vi "5785 Generation.vi"(11 "Frequency (Hz)":dbl=100000000.0 format="%#_6p") -> (0 "error out":errorcluster)   [LabVIEW 2019]
uses:
  <vilib>/userDefined/Silver/nirio_resource_slv.ctl
  <instrlib>/FlexRIO/API/Host/v1/NI FlexRIO/API/Reference Clock Source.ctl
  Common/Original 5785 Example/Host/Upconversion Mode.ctl
  <instrlib>/FlexRIO/API/Host/v1/NI FlexRIO/API/Configure Reference Clock.vi
  <instrlib>/FlexRIO/API/Host/v1/NI FlexRIO/API/Get Property Reference - Fpga Small.vi
  <instrlib>/FlexRIO/API/Host/v1/NI FlexRIO/API/Configure Analog Start Trigger.vi
  <instrlib>/FlexRIO/API/Host/v1/NI FlexRIO/API/Configure Digital Edge Start Trigger.vi
  <instrlib>/FlexRIO/API/Host/v1/NI FlexRIO/API/Configure Immediate Start Trigger.vi
  <vilib>/measure/matone.llb/Extract Single Tone Information N Chan.vi
  <vilib>/measure/maspectr.llb/FFT Power Spectrum and PSD for N Chan.vi
  <vilib>/FPGAPlugInAG/Dynamic/niLvFpga_Close_Dynamic.vi
  <vilib>/rvi/interface/nirviCloseFPGA/nirviCloseFPGA.xnode
  <instrlib>/FlexRIO/API/Host/v1/NI FlexRIO API v1.lvlib
  <resource>/objmgr/niflexrioapiStream.rc
  <vilib>/measure/NI_MAPro.lvlib
  Common/Original 5785 Example/Host/GettingStarted_5785_Host.lvlib
  <instrlib>/FlexRIO/API/Host/v1/NI FlexRIO/API/Read Stream 1D WDT.vi
panel:
  in  "DUC Freq Shift (Hz)":dbl format="%#_4p"
  in  "DDC Freq Shift (Hz)":dbl format="%#_4p"
  in  "IQ Enabled":bool
  in  "DDC Enabled":bool
  in  "processing mode":T1=enum."None, Two Channels"
  out "AO num Samples":i32=160
  in  "waveform config":T2(array[cluster])=[{"Frequency (Hz)"=500000000.0, "Amplitude (V)"=0.2, "Phase (Deg)"=0.0}, {"Frequency (Hz)"=500000000.0, "Amplitude (V)"=0.20000000000000004, "Phase (Deg)"=0.0}] {"Phase (Deg)" format="%.2p"; "Amplitude (V)" format="%0.2p"; "Frequency (Hz)" format="%0.2p"}
  in  "reference clock source":T3 items=["Default", "Onboard", "PXI_Clk10", "External", "None", "Baseboard Reference"]
  in  "Update Waveform":bool caption="Download AO Waveforms"
  out "Sample Rate":dbl=3200000000.0 format="%#_6p"
  in  "ADC Interleaving Factor":i32=1 min=0 max=2 step=1
  in  "AI num samples":u64=320 step=32
  in  "AI channels":string="AI0,AI1"
  out "Device Power":dbl(slide)=32.59 scale=-1.0..58.0 scale format="%#_3p"
  out "FPGA Temperature":dbl(slide)=48.0 scale=0.0..100.0 scale format="%#_3p"
  in  "Trigger Type":enum32{"Immediate", "Analog", "Digital"}(tab)
  in  "trigger channel":string="AI0"
  in  "rising edge?":bool=TRUE
  in  "level (V)":dbl format="%#_3p"
  in  "hysteresis (V)":dbl=0.01 format="%#_3p"
  in  "digital trigger source":string(combo)
  in  "stop":bool
  in  "Bitfile path":path=path "C:/Repos/bsherman-sandbox/CogRF/5785 Measurements/Common/Original 5785 Example/FPGA Bitfiles/PXIe_5785_KU060.lvbitx"
  in  "Waveform Tab Control":T4(tab)
  out "Waveform Graph":waveform(dbl)[](graph)=[{"t0"=timestamp(0 s since 1904-01-01), "dt"=3.125e-10, "Y"=array[320 elements]}, {"t0"=timestamp(0 s since 1904-01-01), "dt"=3.125e-10, "Y"=array[320 elements]}]
  out "FFT":cluster{"f0":dbl, "df":dbl, "magnitude":dbl[]}[](graph)=[{"f0"=0.0, "df"=10000000.0, "magnitude"=[-82.80063413529373, -79.42075070514161, -79.66654847580517, -84.51801585564033, -82.30375380409255, -84.06983083569486, -85.66588756329017, -81.93454044371977, -82.7334518284433, -90.8972761146736, -87.61278142747294, -104.61353149769258, -96.28538776427862, -95.10865239905246, -100.56521482666498, -91.42478181315082, -87.70246288546254, -96.15482624965125, -83.85755926546608, -89.20973033468074, -90.22419818568508, -98.99668681361555, -98.60506381140829, -93.29284897866715, -83.85257693765564, -82.90006467726401, -83.45941426572493, -80.25008158521148, -79.93161770011034, -79.54616931592298, -81.30831360852552, -89.3926211554797, -85.88224547986444, -82.87485908353914, -81.93656330640073, -79.20811557500818, -79.33127118879915, -83.00000028590416, -90.00021633457037, -88.94291208193506, -94.81520575658656, -89.72483865287286, -90.03506772196766, -88.10479845296439, -84.61607135685057, -84.72807586779753, -82.3263452971978, -82.71547656878712, -95.58083173506547, -88.61789584075763, -86.68540478159909, -83.07923596382108, -82.7659009857978, -91.87050343873932, -84.66676602771557, -79.67758660366972, -79.03719798485804, -86.91335832284452, -99.97611534229983, -92.79230181046542, -87.01921960736439, -83.08071759168135, -83.5536303116052, -91.69363274102763, -88.41514807099949, -84.10637487787747, -82.44488027320298, -85.08159037151373, -86.04882507196643, -90.13991844124908, -94.82822338029456, -97.06431232929042, -99.63177607215952, -87.79637869645369, -90.10079393416046, -91.82607525621145, -92.62007187200066, -97.8504266754619, -86.1258854333692, -86.25934378904303, -102.59108879099308, -90.0771213920622, -82.32664139003381, -80.78431775305042, -91.50907884320321, -87.95306054419447, -85.57843269559798, -93.04673637457378, -83.30460156673297, -82.19833423896098, -83.5215038947126, -96.02648947107404, -87.65556995900711, -84.70085134292157, -88.22032498756884, -103.07939027252586, -108.02210671738155, -86.99055305132113, -88.32179529969324, -90.31615125476408, -84.97901674920863, -83.09883311475267, -84.95671844316507, -85.53395021586064, -90.81842173967111, -93.68611641670468, -84.452817075586, -79.89507522416633, -81.39102595505449, -81.52404503339568, -80.48337477433137, -87.87345095289177, -84.30670527149636, -83.09195779094782, -84.84695356438543, -91.72645233073027, -88.3626801362871, -90.81004429684762, -87.45943061943689, -90.26039906388364, -90.45094731656192, -87.51778499753328, -80.36998792980968, -80.90573377879318, -93.04936796269288, -86.4132138459746, -93.72990076985027, -83.6736250082015, -83.99855859467331, -89.3953164516118, -83.81187005387955, -87.49573067759147, -84.23606489302381, -83.16298492778144, -87.1194948264914, -90.99142642379402, -93.24764967458385, -88.63527313931499, -102.49413654042559, -90.66118161659553, -92.25646188435081, -80.9110366436795, -83.55380603169064, -81.01720552981077, -84.3777210205706, -90.31462939121568, -98.00294051178642, -95.60338217280496, -96.72557339603003, -85.0751852630811, -82.8903033043814, -96.97498517828193, -84.68377849718097, -81.38086551188258, -85.79249998005481, -87.70913834096886, -93.06972137639319, -97.21572279595078, -95.86294146140558, -83.02562226491523]}, {"f0"=0.0, "df"=10000000.0, "magnitude"=[-64.78931072488608, -67.73528418446969, -87.87073015272404, -81.21018837283968, -80.84885582450725, -84.81155481886637, -87.62283168377273, -82.75665314945999, -83.33624895976874, -85.00935247454665, -90.01344899655619, -85.4168344363582, -93.77738192601578, -88.78723575716211, -80.89555662638084, -77.40445430057734, -83.04964925849828, -92.69503327640547, -85.33098178751953, -84.21675735932456, -94.4286131086485, -84.18522106861258, -84.126502324857, -86.19640568640202, -87.43382048150457, -90.03983448655742, -83.08248688320506, -77.13727685427946, -78.52531931117574, -82.27551749332419, -87.38788534435882, -86.09983091368706, -85.9317566084158, -93.3787076269555, -90.43872921677129, -85.03312454760936, -93.48170429395404, -96.606174398692, -84.54369527641475, -80.1677671442906, -82.28530110524787, -83.58711730195151, -82.75878126450083, -83.35504507620462, -86.06919066007586, -101.11499708979125, -91.71195220747622, -83.56465114361383, -79.52150767688725, -79.96380630019732, -91.4050434521125, -83.48310537201712, -81.73837395801057, -87.51107955857, -89.7119800165195, -81.42579926328145, -79.58251225051853, -83.06097697370845, -88.76806290183217, -82.58018678115121, -80.02121778615148, -82.16358703095486, -86.62565282274939, -99.28526757279388, -94.99464094911238, -90.72589358589816, -88.18693112559416, -79.36875927098997, -79.20171789778858, -83.94202736003771, -105.55799216649051, -83.12357738578754, -82.44879182647495, -86.27524307450246, -88.28406841938097, -81.19621273977118, -83.87578114234637, -88.5269238392554, -84.41995093103635, -85.35505706638736, -84.92519624410147, -81.97290731818995, -82.8267656339678, -82.54032928873265, -86.79451163672385, -88.78654921566789, -81.32210725089064, -82.90482422458243, -86.60048725134602, -86.831633705738, -85.73730495943633, -83.52042201274215, -88.5297416330032, -95.45249595410544, -97.22152770134748, -96.95556150404856, -88.61342235545409, -87.4643325338421, -80.28275240840776, -78.03157534185394, -82.88175719417588, -93.39877945578407, -99.90212582359797, -85.2979962460108, -86.22850917558934, -86.56007545671977, -106.08884169104671, -85.38285757853984, -88.82365520443673, -95.23608231604402, -88.02164481094161, -93.28020634203888, -95.02500522087377, -86.86550910566638, -106.28569332849621, -94.87588536988524, -99.26453951216462, -87.13456076973338, -81.47213984719738, -78.75854685696707, -78.65463828489014, -82.49223582204748, -97.5364174442158, -95.08344525435209, -87.23974238111994, -90.45342808286607, -93.02309157165219, -87.82563643069052, -89.6611716765326, -81.02521384215505, -82.27408401978239, -86.2519183286075, -87.26967132350863, -82.01085019692505, -80.81243914798475, -82.27515501657854, -86.70178876516077, -79.23742538829981, -79.68471508937189, -84.67318859876387, -82.27227290640813, -76.20448461790832, -78.88688649209806, -90.59786677274529, -92.25114985663237, -91.460612834368, -91.26343664898255, -82.08959989225445, -86.11895874760603, -95.1222735792313, -86.44672739810025, -78.83968447685616, -79.23597642096348, -87.541546971985, -88.11663602685513, -84.13844747103789, -85.96460534965021, -88.21924098304329, -84.25148312866752, -76.29493493073782]}] caption="Waveform Graph"
  out "detected frequencies":dbl[](array[numeric])=[555552707.7834543, 1412702117.9341562] format="%_4p"
  out "AO Out":waveform(dbl)[](graph)=[{"t0"=timestamp(0 s since 1904-01-01), "dt"=3.125e-10, "Y"=[0.0, 0.16629392246050906, 0.1847759065022574, 0.03901806440322561, -0.1414213562373095, -0.19615705608064604, -0.07653668647301802, 0.11111404660392049, 0.2, 0.11111404660392035, -0.07653668647301787, -0.19615705608064607, -0.14142135623730956, 0.03901806440322578, 0.18477590650225734, 0.16629392246050892, 0.0, -0.16629392246050909, -0.18477590650225734, -0.03901806440322547, 0.14142135623730956, 0.196157056080646, 0.07653668647301785, -0.11111404660392055, -0.19999999999999996, -0.11111404660392023, 0.07653668647301798, 0.19615705608064604, 0.1414213562373094, -0.03901806440322589, -0.18477590650225728, -0.1662939224605088, 5.551115123125783e-17, 0.16629392246050909, 0.18477590650225723, 0.03901806440322533, -0.14142135623730945, -0.19615705608064585, -0.07653668647301788, 0.11111404660392057, 0.1999999999999999, 0.11111404660392012, -0.07653668647301798, -0.196157056080646, -0.14142135623730936, 0.03901806440322589, 0.18477590650225725, 0.16629392246050878, -2.7755575615628914e-17, -0.16629392246050906, -0.18477590650225725, -0.03901806440322536, 0.14142135623730942, 0.19615705608064593, 0.07653668647301794, -0.11111404660392066, -0.1999999999999999, -0.11111404660392014, 0.07653668647301792, 0.19615705608064604, 0.14142135623730945, -0.039018064403225916, -0.18477590650225728, -0.1662939224605088, 0.0, 0.16629392246050914, 0.18477590650225728, 0.03901806440322533, -0.14142135623730945, -0.19615705608064596, -0.07653668647301792, 0.11111404660392063, 0.1999999999999999, 0.11111404660392017, -0.07653668647301792, -0.1961570560806461, -0.14142135623730945, 0.039018064403226, 0.18477590650225728, 0.1662939224605088, 0.0, -0.1662939224605092, -0.18477590650225728, -0.039018064403225305, 0.14142135623730945, 0.196157056080646, 0.07653668647301792, -0.11111404660392071, -0.1999999999999999, -0.11111404660392012, 0.07653668647301792, 0.19615705608064615, 0.14142135623730945, -0.039018064403226055, -0.18477590650225728, -0.1662939224605088, 0.0, 0.16629392246050925, 0.18477590650225728, 0.039018064403225305, -0.14142135623730945, -0.19615705608064601, -0.07653668647301792, 0.11111404660392074, 0.1999999999999999, 0.11111404660392014, -0.07653668647301792, -0.1961570560806461, -0.14142135623730945, 0.03901806440322597, 0.18477590650225728, 0.1662939224605088, 0.0, -0.16629392246050914, -0.18477590650225728, -0.03901806440322539, 0.14142135623730945, 0.196157056080646, 0.07653668647301792, -0.1111140466039206, -0.1999999999999999, -0.11111404660392023, 0.07653668647301792, 0.19615705608064604, 0.14142135623730945, -0.03901806440322583, -0.18477590650225728, -0.16629392246050886, 0.0, 0.16629392246050909, 0.18477590650225728, 0.03901806440322539, -0.14142135623730945, -0.19615705608064593, -0.07653668647301792, 0.1111140466039206, 0.1999999999999999, 0.11111404660392019, -0.07653668647301792, -0.19615705608064607, -0.14142135623730945, 0.039018064403225944, 0.18477590650225728, 0.1662939224605088, 0.0, -0.16629392246050914, -0.18477590650225728, -0.03901806440322533, 0.14142135623730945, 0.19615705608064596, 0.07653668647301792, -0.11111404660392063, -0.1999999999999999, -0.11111404660392017, 0.07653668647301792, 0.1961570560806461, 0.14142135623730945, -0.039018064403226, -0.18477590650225728, -0.1662939224605088]}, {"t0"=timestamp(0 s since 1904-01-01), "dt"=3.125e-10, "Y"=[0.0, 0.16629392246050909, 0.1847759065022574, 0.03901806440322561, -0.1414213562373095, -0.19615705608064612, -0.07653668647301798, 0.11111404660392046, 0.20000000000000004, 0.11111404660392046, -0.076536686473018, -0.19615705608064612, -0.1414213562373095, 0.03901806440322561, 0.1847759065022574, 0.1662939224605091, 0.0, -0.166293922460509, -0.1847759065022574, -0.03901806440322575, 0.1414213562373095, 0.1961570560806461, 0.07653668647301802, -0.11111404660392044, -0.2, -0.11111404660392044, 0.07653668647301787, 0.1961570560806461, 0.14142135623730956, -0.03901806440322575, -0.18477590650225734, -0.16629392246050897, 0.0, 0.16629392246050903, 0.18477590650225734, 0.03901806440322558, -0.14142135623730956, -0.196157056080646, -0.07653668647301785, 0.11111404660392044, 0.19999999999999996, 0.11111404660392034, -0.07653668647301798, -0.196157056080646, -0.1414213562373094, 0.039018064403225666, 0.18477590650225728, 0.16629392246050895, -5.551115123125783e-17, -0.166293922460509, -0.18477590650225723, -0.039018064403225555, 0.14142135623730945, 0.19615705608064596, 0.07653668647301788, -0.11111404660392041, -0.1999999999999999, -0.11111404660392037, 0.07653668647301798, 0.196157056080646, 0.14142135623730936, -0.03901806440322561, -0.18477590650225725, -0.16629392246050897, 2.7755575615628914e-17, 0.16629392246050897, 0.18477590650225725, 0.03901806440322564, -0.14142135623730942, -0.19615705608064601, -0.07653668647301794, 0.11111404660392041, 0.1999999999999999, 0.11111404660392041, -0.07653668647301792, -0.19615705608064601, -0.14142135623730945, 0.03901806440322564, 0.18477590650225728, 0.16629392246050897, 0.0, -0.16629392246050897, -0.18477590650225728, -0.03901806440322564, 0.14142135623730945, 0.19615705608064601, 0.07653668647301792, -0.11111404660392041, -0.1999999999999999, -0.11111404660392041, 0.07653668647301792, 0.19615705608064601, 0.14142135623730945, -0.03901806440322564, -0.18477590650225728, -0.16629392246050897, 0.0, 0.16629392246050897, 0.18477590650225728, 0.03901806440322564, -0.14142135623730945, -0.19615705608064601, -0.07653668647301792, 0.11111404660392041, 0.1999999999999999, 0.11111404660392041, -0.07653668647301792, -0.19615705608064601, -0.14142135623730945, 0.03901806440322564, 0.18477590650225728, 0.16629392246050897, 0.0, -0.16629392246050897, -0.18477590650225728, -0.03901806440322564, 0.14142135623730945, 0.19615705608064601, 0.07653668647301792, -0.11111404660392041, -0.1999999999999999, -0.11111404660392041, 0.07653668647301792, 0.19615705608064601, 0.14142135623730945, -0.03901806440322564, -0.18477590650225728, -0.16629392246050897, 0.0, 0.16629392246050897, 0.18477590650225728, 0.03901806440322564, -0.14142135623730945, -0.19615705608064601, -0.07653668647301792, 0.11111404660392041, 0.1999999999999999, 0.11111404660392041, -0.07653668647301792, -0.19615705608064601, -0.14142135623730945, 0.03901806440322564, 0.18477590650225728, 0.16629392246050897, 0.0, -0.16629392246050897, -0.18477590650225728, -0.03901806440322564, 0.14142135623730945, 0.19615705608064601, 0.07653668647301792, -0.11111404660392041, -0.1999999999999999, -0.11111404660392041, 0.07653668647301792, 0.19615705608064601, 0.14142135623730945, -0.03901806440322564, -0.18477590650225728, -0.16629392246050897]}] caption="Waveform Graph"
  out "Limit (W)":dbl=58.0
  out "Power (W)":dbl=32.59
  out "Limit (C)":dbl=96.0
  out "Temp (C)":dbl=48.0 format="%#_4p"
  in  "RIO Device":T5="5785_00"
  # "Overview: Configure an acquisition for a FlexRIO target and transfer the data to the host using the FlexRIO Host API.  Loop an output waveform\nRequirements: FlexRIO\nInstructions: \n 1. Loop AI channels back to AO channels using SMA cables\n 2. Select the RIO Device that corresponds to the FlexRIO target. \n 3. Select the bitfile path that corresponds to your device\n 4. Optionally configure the clocking, stream, and trigger. \n 5. Run the VI"
  # "Resource Configuration"
  # "Clocking configuration"
  # "Input Waveform Configuration"
  # "Device Monitoring"
  # "Output Waveform Configuration"
  # "Digital Upconverter Configuration"
  # "Frequency (Hz)"
  # "Amplitude (V)"
  # "Phase (Deg)"
  # "AO 0"
  # "AO 1"
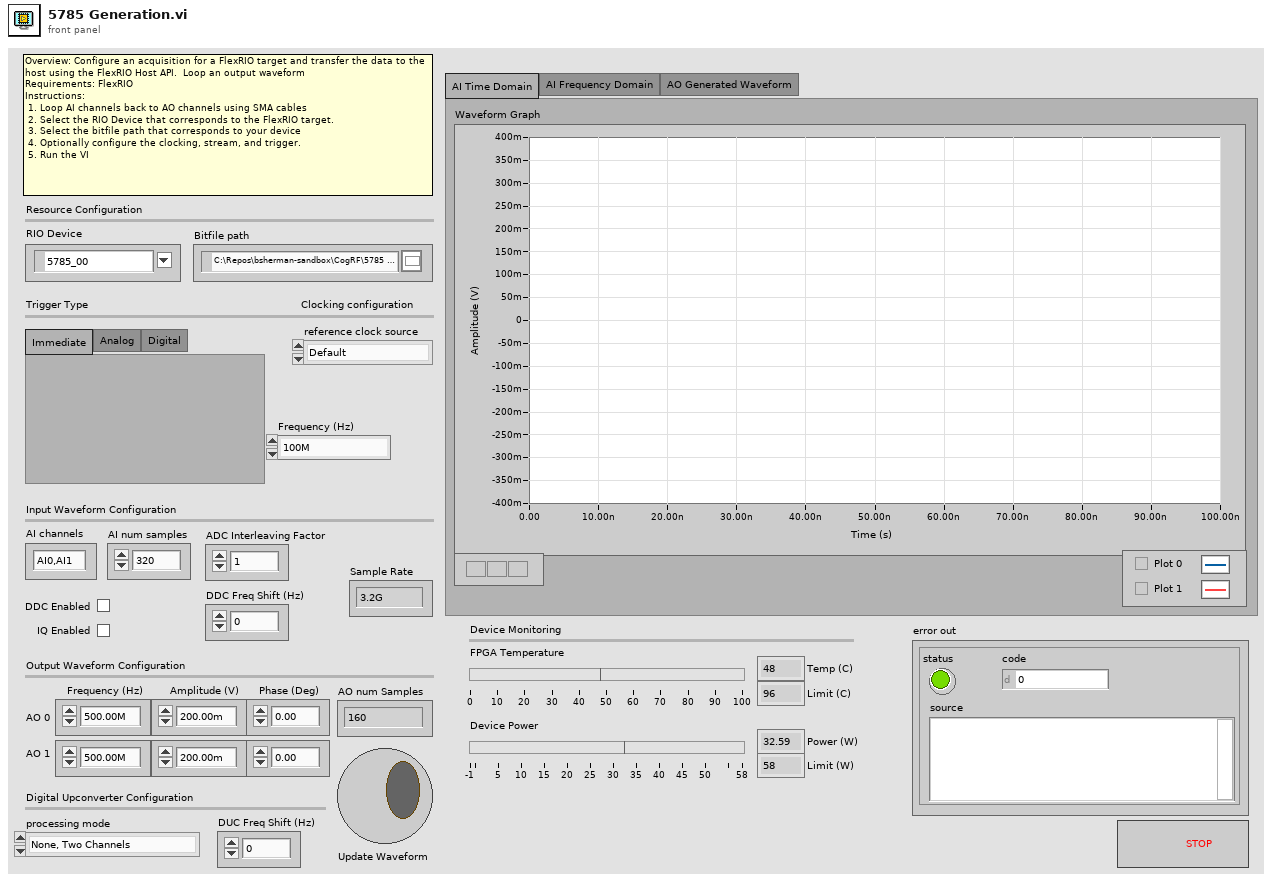
[diagram p1: front panel]
types:
  T1 = typedef "GettingStarted_5785_Host.lvlib/Upconversion Mode.ctl" = enum16{"None, One Channel", "None, Two Channels", "FPGA-only, One Channel", "DAC and FPGA, One Channel", "DAC-only, One Channel"}
  T2 = cluster{"Frequency (Hz)":dbl, "Amplitude (V)":dbl, "Phase (Deg)":dbl}[]
  T3 = typedef "NI FlexRIO API v1.lvlib/Reference Clock Source.ctl" = i32
  T4 = enum32{"AI Time Domain", "AI Frequency Domain", "AO Generated Waveform"}
  T5 = typedef "nirio_resource_slv.ctl" = tag
  T6 = cluster{"averaging mode":enum16{"No averaging", "Vector averaging", "RMS averaging", "Peak hold"}, "weighting mode":enum16{"Linear", "Exponential"}, "number of averages":u32}
  T7 = cluster{"Frequency (Hz)":dbl, "Amplitude (V)":dbl, "Phase (Deg)":dbl}
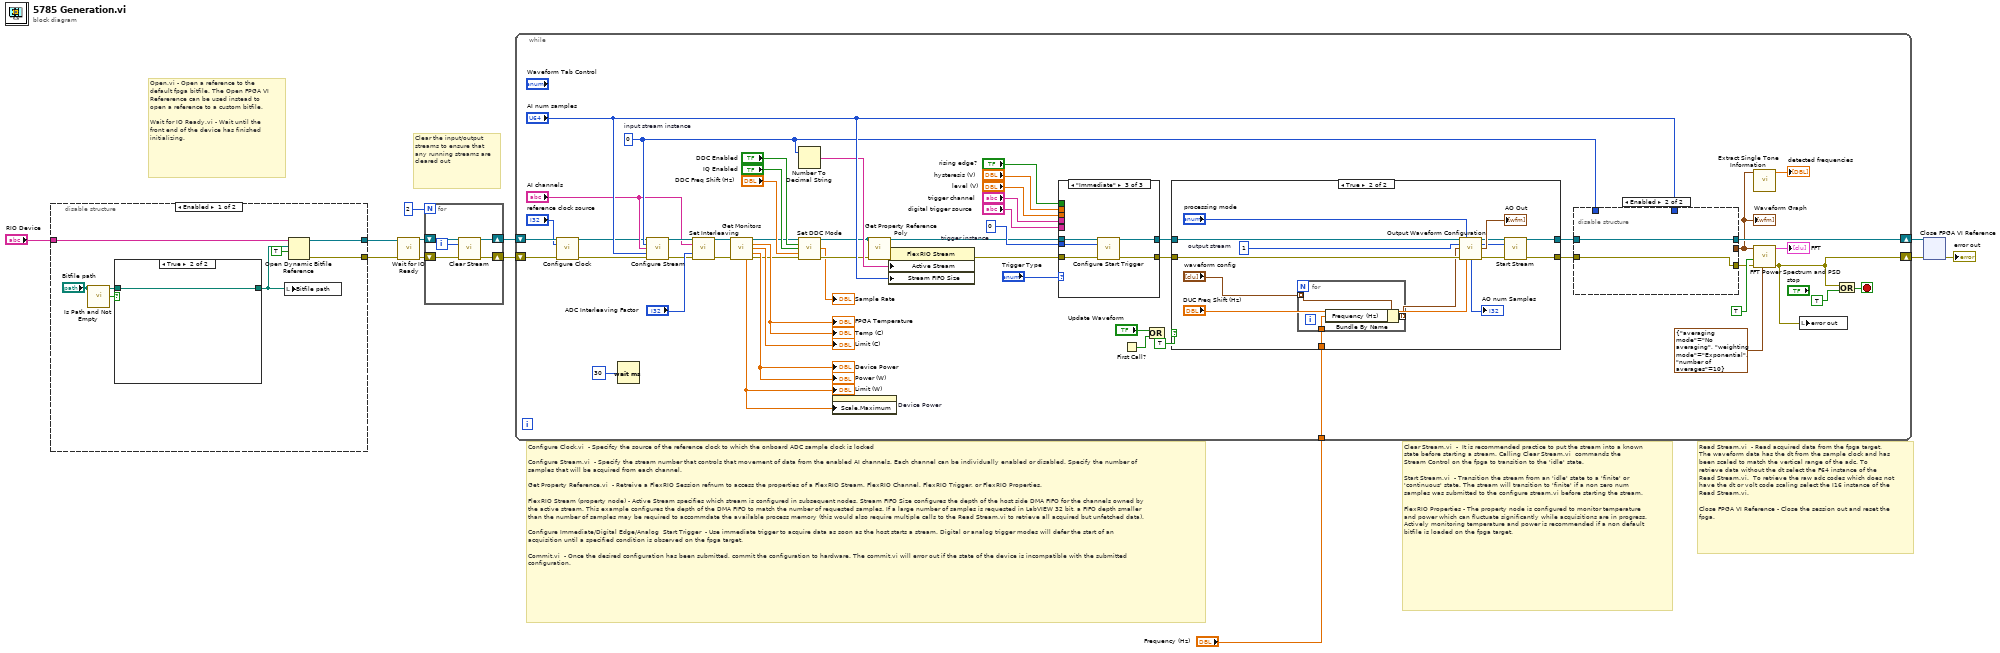
[diagram p0: block diagram]
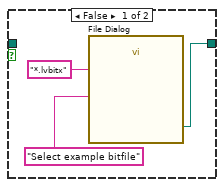
[diagram p2: hidden frame]
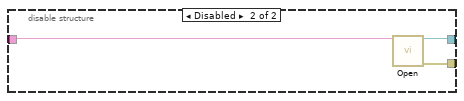
[diagram p3: hidden frame]
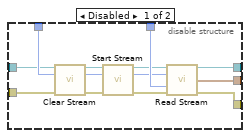
[diagram p4: hidden frame]
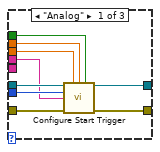
[diagram p6: hidden frame]
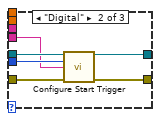
[diagram p7: hidden frame]
diagram:
  # "Clear the input/output\nstreams to ensure that\nany running streams are cleared out"
  # "Read Stream.vi  - Read acquired data from the fpga target. The waveform data has the dt from the sample clock and has been scaled to match the vertical range of the adc. To retrieve data without the dt select the F64 instance of the Read Stream.vi.  To retrieve the raw adc codes which does not have the dt or volt code scaling select the I16 instance of the Read Stream.vi.  \n\nClose FPGA VI Reference - Close the session out and reset the fpga."
  # "Clear Stream.vi  -  It is recommended practice to put the stream into a known state before starting a stream. Calling Clear Stream.vi  commands the Stream Control on the fpga to transition to the 'idle' state.\n\nStart Stream.vi  - Transition the stream from an 'idle' state to a 'finite' or 'continuous' state. The stream will transition to 'finite' if a non zero num samples was submitted to the configure stream.vi before starting the stream.  \n\nFlexRIO Properties - The property node is configured to monitor temperature and power which can fluctuate significantly while acquisitions are in progress. Actively monitoring temperature and power is recommended if a non default bitfile is loaded on the fpga target."
  # "Configure Clock.vi  - Specifcy the source of the reference clock to which the onboard ADC sample clock is locked\n\nConfigure Stream.vi  - Specify the stream number that controls that movement of data from the enabled AI channels. Each channel can be individually enabled or disabled. Specify the number of samples that will be acquired from each channel. \n\nGet Property Reference.vi  - Retreive a FlexRIO Session refnum to access the properties of a FlexRIO Stream, FlexRIO Channel, FlexRIO Trigger, or FlexRIO Properties.\n\nFlexRIO Stream (property node) - Active Stream specifies which stream is configured in subsequent nodes. Stream FIFO Size configures the depth of the host side DMA FIFO for the channels owned by the active stream. This example configures the depth of the DMA FIFO to match the number of requested samples. If a large number of samples is requested in LabVIEW 32 bit, a FIFO depth smaller than the number of samples may be required to accommdate the available process memory (this would also require multiple calls to the Read Stream.vi to retrieve all acquired but unfetched data). \n\nConfigure Immediate/Digital Edge/Analog  Start Trigger  - Use immediate trigger to acquire data as soon as the host starts a stream. Digital or analog trigger modes will defer the start of an acquisition until a specified condition is observed on the fpga target. \n\nCommit.vi  - Once the desired configuration has been submitted, commit the configuration to hardware. The commit.vi will error out if the state of the device is incompatible with the submitted configuration."
  # "Open.vi - Open a reference to the default fpga bitfile. The Open FPGA VI Refererence can be used instead to open a reference to a custom bitfile.\n\nWait for IO Ready.vi - Wait until the front end of the device has finished initializing."
  n1 = disable-structure shown="Enabled" {
    disable-tunnel: [w19 w26] -> w11
    disable-tunnel: [w18 w25] -> w10
    disable-tunnel: "RIO Device" -> [w17 w24]
    frame Enabled {
      n2 = call <vilib>:"Is Path and Not Empty.vi"("path"="Bitfile path") -> ("Is Path and Not Empty?"=w14:bool)  [unwired: 4 in]
      n3 = case shown="True" w14 {
        tunnel: "Bitfile path" -> [_ w23]
        tunnel: [w21 w23] -> w13
        frame False {
          n4 = call "File Dialog"("prompt"="Select example bitfile", "pattern (all files)"="*.lvbitx") -> ("selected path"=w21:path)  [unwired: 10 in, 3 out]
        }
        frame True {
        }
      }
      n5 = local write "Bitfile path"(w13) -> ()
      n6 = Open Dynamic Bitfile Reference(0:w17, 1:w13, 2:TRUE ("Run When Loaded")) -> (5:w18:refnum<k20>, 8:w19:errorcluster)  [unwired: 2 in]
    }
    frame Disabled {
      n7 = call <instrlib>:"Open.vi"("RIO Device"=w24) -> ("fpga interface out"=w25:refnum<k20>, "error out"=w26:errorcluster)  [unwired: 13 in]
    }
  }
  n8 = call <instrlib>:"Wait for IO Ready.vi"("fpga interface in"=w10, "error in"=w11) -> ("fpga interface out"=w6:refnum<k20>, "error out"=w5:errorcluster)  [unwired: 10 in, 2 out]
  n9 = for {
    N: 2 -> [_]
    shift-right: [w28] -> w3
    shift-left: w6 -> [w31]
    shift-right: [w29] -> w4
    shift-left: w5 -> [w30]
    i -> [w27]
    n10 = call <instrlib>:"Clear Stream.vi"("fpga interface in"=w31, "stream instance"=w27, "error in"=w30) -> ("fpga interface out"=w28:refnum<k20>, "error out"=w29:errorcluster)  [unwired: 10 in, 1 out]
  }
  n11 = while {
    shift-right: [w48] -> w7
    shift-left: w4 -> [w86]
    shift-right: [w84] -> w8
    shift-left: w3 -> [w85]
    tunnel: "Frequency (Hz)" -> [w34]
    stop <- w56 stop-if-true
    w75 = u32 0  # trigger instance
    w71 = u32 0  # input stream instance
    n12 = call-poly <instrlib>:"Configure Clock.vi"("fpga interface in"=w85, "reference clock source"="reference clock source", "error in"=w86) -> ("fpga interface out"=w52:refnum<k20>, "error out"=w79:errorcluster)  [unwired: 11 in]
    n13 = Wait (ms)(milliseconds to wait=u32 30) -> ()  [unwired: 1 out]
    n14 = call <instrlib>:"Configure Stream.vi"("fpga interface in"=w52, "stream instance"=w71, "channels enabled"="AI channels", "num samples"="AI num samples", "error in"=w79) -> ("fpga interface out"=w69:refnum<k20>, "error out"=w67:errorcluster)  [unwired: 7 in, 2 out]
    n15 = call "Set Interleaving.vi"("fpga interface in"=w69, "AI channels enabled"="AI channels", "ADC Interleaving Factor"="ADC Interleaving Factor", "error in (no error)"=w67) -> ("fpga interface out"=w54:refnum<k20>, "error out"=w53:errorcluster)  [unwired: 10 in]
    n16 = call "Get Monitors.vi"("fpga interface in"=w54, "error in (no error)"=w53) -> ("fpga interface out"=w40:refnum<k20>, "FPGA Temperature (C)"=→"Temp (C)" →"FPGA Temperature":dbl, "Temperature Limit (C)"=→"Limit (C)":dbl, "Total Power (W)"=→"Power (W)" →"Device Power":dbl, "Power Limit (W)"=w61:dbl, "error out"=w39:errorcluster)  [unwired: 8 in]
    "Limit (W)" <- w61
    n17 = Number To Decimal String(number=w71) -> (decimal integer string=w77:string)  [unwired: 1 in]
    n18 = call "Set DDC Mode.vi"("fpga refnum"=w40, "DDC Enabled"="DDC Enabled", "IQ Enabled"="IQ Enabled", "DDC Frequency Shift (Hz)"="DDC Freq Shift (Hz)", "error in (no error)"=w39) -> ("fpga refnum out"=w41:refnum<k20>, "sample rate"=→"Sample Rate":dbl, "error out"=w42:errorcluster)  [unwired: 8 in]
    n19 = property on="Device Power" class="Slide (strict)"("Scale.Maximum"=w61) -> ()  [unwired: 2 in, 2 out]
    n20 = call-poly <instrlib>:"Get Property Reference Poly.vi"("error in (no error)"=w42, "fpga interface in"=w41) -> ("error out"=w66:errorcluster, "property reference"=w65:refnum<k20>)  [unwired: 4 in, 1 out]
    n21 = property class="FlexRIO Stream"(reference=w65, error in=w66, "Active Stream"=w77, "Stream FIFO Size"="AI num samples") -> (error out=w74:errorcluster)  [unwired: 1 out]
    n22 = case shown="\"Immediate\"" "Trigger Type" {
      tunnel: w41 -> [w130 w136 w141]
      tunnel: w74 -> [w129 w135 w140]
      tunnel: [w128 w134 w139] -> w73
      tunnel: [w127 w133 w138] -> w72
      tunnel: w75 -> [w126 w132 w137]
      tunnel: "trigger channel" -> [w125 _ _]
      tunnel: "level (V)" -> [w124 _ _]
      tunnel: "hysteresis (V)" -> [w123 _ _]
      tunnel: "rising edge?" -> [w122 _ _]
      tunnel: "digital trigger source" -> [_ w131 _]
      frame "Analog" {
        n23 = call-poly <instrlib>:"Configure Start Trigger.vi"("fpga interface in"=w130, "level"=w124, "hysteresis"=w123, "rising edge?"=w122, "trigger instance"=w126, "channel"=w125, "error in"=w129) -> ("fpga interface out"=w128:refnum<k20>, "error out"=w127:errorcluster)  [unwired: 6 in, 1 out]
      }
      frame "Digital" {
        n24 = call-poly <instrlib>:"Configure Start Trigger.vi"("fpga interface in"=w136, "trigger instance"=w132, "trigger source"=w131, "error in"=w135) -> ("fpga interface out"=w134:refnum<k20>, "error out"=w133:errorcluster)  [unwired: 9 in, 1 out]
      }
      frame "Immediate" {
        n25 = call-poly <instrlib>:"Configure Start Trigger.vi"("fpga interface in"=w141, "trigger instance"=w137, "error in"=w140) -> ("fpga interface out"=w139:refnum<k20>, "error out"=w138:errorcluster)  [unwired: 10 in, 1 out]
      }
    }
    n26 = First Call?() -> (First Call?: T/F=w35:bool)
    n27 = Or(x="Update Waveform", y=w35) -> ()  [unwired: 1 out]
    n28 = case shown="True" TRUE {
      tunnel: [w103 w118] -> w47
      tunnel: [w102 w117] -> w46
      tunnel: w73 -> [w103 w115]
      tunnel: w72 -> [w102 w114]
      tunnel: w34 -> [_ w104]
      frame False {
      }
      frame True {
        w111 = u32 1  # output stream
        n29 = for {
          tunnel: "waveform config" -> [w121] mode=indexing
          tunnel: [w120] -> w105 mode=indexing
          tunnel: w104 -> [w119]
          n30 = Bundle By Name(cluster=w121, "Frequency (Hz)"=w119) -> (w120:T7)
        }
        n31 = call "Output Waveform Configuration.vi"("Refnum in"=w115, "processing mode"="processing mode", "output stream instance"=w111, "waveform config"=w105, "error in (no error)"=w114, "DUC Frequency Shift"="DUC Freq Shift (Hz)") -> ("Refnum out"=w112:refnum<k20>, "output stream instance out"=w110:u32, "waveforms out"=→"AO Out":waveform(dbl)[], "ao wfm samples"=→"AO num Samples":i32, "error out"=w113:errorcluster)  [unwired: 5 in]
        n32 = call <instrlib>:"Start Stream.vi"("fpga interface in"=w112, "stream instance"=w110, "error in"=w113) -> ("fpga interface out"=w118:refnum<k20>, "error out"=w117:errorcluster)  [unwired: 10 in, 1 out]
      }
    }
    n33 = disable-structure shown="Enabled" {
      disable-tunnel: [w99 w101] -> w84
      disable-tunnel: "AI num samples" -> [w98 _]
      disable-tunnel: w71 -> [w97 _]
      disable-tunnel: [w92 w100] -> w57
      disable-tunnel: [w89 _] -> w51
      disable-tunnel: w47 -> [w88 w101]
      disable-tunnel: w46 -> [w87 w100]
      frame Disabled {
        n34 = call <instrlib>:"Clear Stream.vi"("fpga interface in"=w88, "stream instance"=w97, "error in"=w87) -> ("fpga interface out"=w96:refnum<k20>, "stream instance out"=w95:u32, "error out"=w94:errorcluster)  [unwired: 10 in]
        n35 = call <instrlib>:"Start Stream.vi"("fpga interface in"=w96, "stream instance"=w95, "error in"=w94) -> ("fpga interface out"=w91:refnum<k20>, "stream instance out"=w93:u32, "error out"=w90:errorcluster)  [unwired: 10 in]
        n36 = call-poly <instrlib>:"Read Stream.vi"("fpga interface in"=w91, "stream instance"=w93, "samples"=w98, "error in"=w90) -> ("fpga interface out"=w99:refnum<k20>, "read data"=w89:waveform(dbl)[], "error out"=w92:errorcluster)  [unwired: 7 in, 2 out]
      }
      frame Enabled {
      }
    }
    "Waveform Graph" <- w51
    n37 = call-poly <vilib>:"Extract Single Tone Information.vi"("time signals in"=w51) -> ("detected frequencies"=→"detected frequencies":dbl[])  [unwired: 5 in, 5 out]
    n38 = call-poly <vilib>:"FFT Power Spectrum and PSD.vi"("averaging parameters"=T6 {"averaging mode"=enum."No averaging", "weighting mode"=enum."Exponential", "number of averages"=10}, "error in (no error)"=w57, "dB On (F)"=TRUE, "time signals"=w51) -> ("error out"=w48:errorcluster, "Power Spectrum / PSD"=→"FFT":cluster{"f0":dbl, "df":dbl, "magnitude":dbl[]}[])  [unwired: 4 in, 2 out]
    n39 = local write "error out"(w48) -> ()
    n40 = Or(x=w48, y=TRUE) -> (x .or. y?=w56:bool)
  }
  n41 = xnode "Close FPGA VI Reference"("FPGA VI Reference In"=w8, "error in"=w7) -> ("error out"=→"error out":errorcluster)
